vi "uObserver_Set_Broker.vi"(8 "error in (no error)":errorcluster, 10 "Broker's Transport":refnum<class "uTransport_uActor.lvclass">, 11 "uObserver in":refnum<class "uObserver.lvclass">) -> (0 "error out":errorcluster, 3 "uObserver out":refnum<class "uObserver.lvclass">)   [LabVIEW 2023, in "uLib.lvlib" / "uObserver.lvclass"]
doc: "Pass in the transport of the broker to which this observer is supposed to register to. If this is invoked by the caller prior to launching the actor, an observer with a default non-overridden behavior will not ignore the actual application's broker or the context broker, and will just stick to what has been provided.\n\nDo NOT use this method in conjunction with the Set_DoesOwnBroker accessor method."
uses:
  uObserver.lvclass
  uTransport/uTransport_uActor/uTransport_uActor.lvclass
  uObserver.lvclass/uObserver.ctl
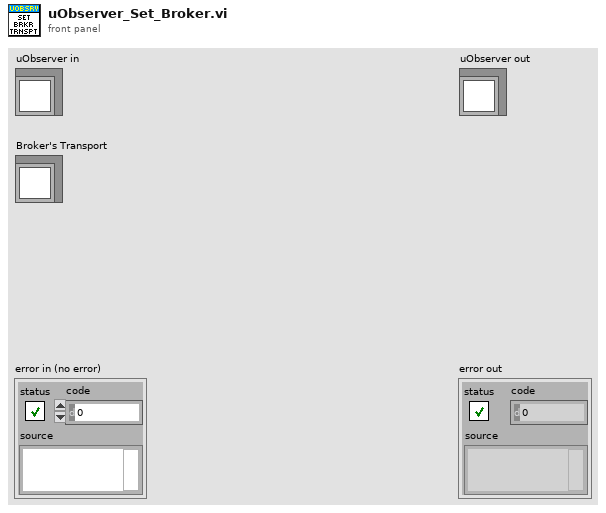
[diagram p1: front panel]
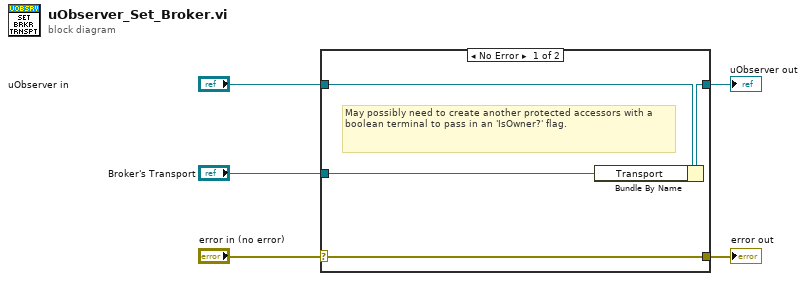
[diagram p0: block diagram]
diagram:
  n1 = case shown="No Error" "error in (no error)" {
    selector: "error in (no error)" -> [w9 w10]
    tunnel: [w9 w10] -> w4
    tunnel: [w7 w11] -> w2
    tunnel: "uObserver in" -> [w8 w11]
    tunnel: "Broker's Transport" -> [w6 _]
    frame No Error {
      # "May possibly need to create another protected accessors with a boolean terminal to pass in an 'IsOwner?' flag."
      n2 = Bundle By Name(cluster=w8, "Transport"=w6) -> (w7:refnum<class "uObserver.lvclass">)
    }
    frame Error {
    }
  }
  "error out" <- w4
  "uObserver out" <- w2
